vi "Fit VI window to Visible Content.vi"(4 "error in (no error)":errorcluster, 6 "border spacing (2 px)":i32=2, 7 "VI Ref (calling VI)":refnum<vi>) -> (0 "error out":errorcluster, 3 "dup VI Ref":refnum<vi>)   [LabVIEW 2017]
doc: "This utility will fit (resize and center) a VI (defined by the \"VI Ref\" input) about the all of the Front Panel object. It will add a border defined by border spacing in units of pixels. If no VI Reference is passed in, it will operate on the calling VI."
uses:
  <userlib>/_OpenG.lib/appcontrol/appcontrol.llb/Close Generic Object Refnum (Array)__ogtk.vi
panel:
  # "Fit VI window to Content.vi\n\nFits a VI's front panel window to its FP Contents.\n\nPlease visit http://www.OpenG.org to learn about the\nOpen Source LabVIEW software movement.\n\nNOTICE -- YOU MUST LEAVE THIS NOTICE IN PLACE.  PER THE TERMS OF THE LICENSE BELOW, YOU MAY SUBLICENSE THIS SOFTWARE \nIN ANY WAY THAT DOES NOT CONFLICT WITH THIS LICENSE.\n\n### BSD License (http://www.opensource.org/licenses/bsd-license.php) Begin ###\n \nCopyright (c) 2002-2004, Jim Kring <jim@jimkring.com>\nCopyright (c) 2002, Cal-Bay Systems, Inc. <info@calbay.com>\n\nAll rights reserved.\n\nRedistribution and use in source and binary forms, with or without modification, are permitted provided that the following conditions are met:\n\n    * Redistributions of source code must retain the above copyright notice, this list of conditions and the following disclaimer.\n    * Redistributions in binary form must reproduce the above copyright notice, this list of conditions and the following disclaimer in the \n       documentation and/or other materials provided with the distribution.\n    * Neither the name of SciWare, James Kring, Inc., nor the names of its contributors may be used to endorse or promote products derived \n       from this software without specific prior written permission.\n\nTHIS SOFTWARE IS PROVIDED BY THE COPYRIGHT HOLDERS AND CONTRIBUTORS \"AS IS\" AND ANY EXPRESS OR IMPLIED WARRANTIES, \nINCLUDING, BUT NOT LIMITED TO, THE IMPLIED WARRANTIES OF MERCHANTABILITY AND FITNESS FOR A PARTICULAR PURPOSE ARE \nDISCLAIMED. IN NO EVENT SHALL THE COPYRIGHT OWNER OR CONTRIBUTORS BE LIABLE FOR ANY DIRECT, INDIRECT, INCIDENTAL,\n SPECIAL, EXEMPLARY, OR CONSEQUENTIAL DAMAGES (INCLUDING, BUT NOT LIMITED TO, PROCUREMENT OF SUBSTITUTE GOODS OR \nSERVICES; LOSS OF USE, DATA, OR PROFITS; OR BUSINESS INTERRUPTION) HOWEVER CAUSED AND ON ANY THEORY OF LIABILITY, \nWHETHER IN CONTRACT, STRICT LIABILITY, OR TORT (INCLUDING NEGLIGENCE OR OTHERWISE) ARISING IN ANY WAY OUT OF THE USE \nOF THIS SOFTWARE, EVEN IF ADVISED OF THE POSSIBILITY OF SUCH DAMAGE.\n\n### BSD License End ###"
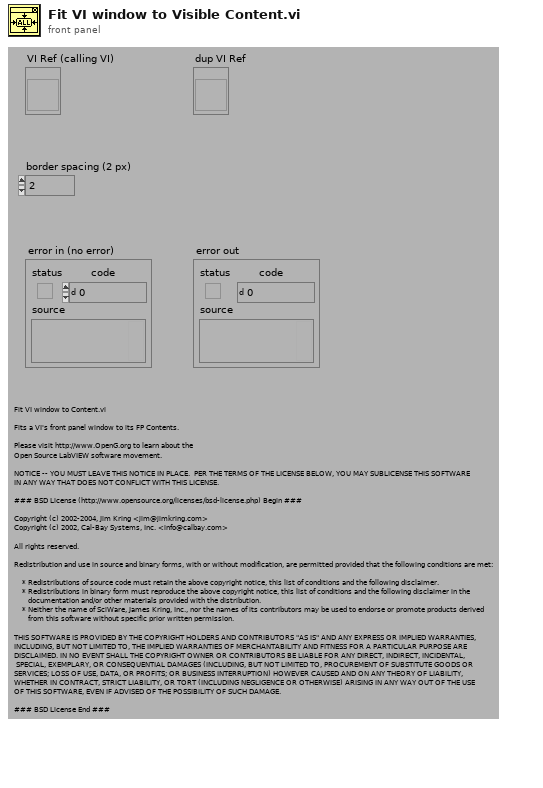
[diagram p1: front panel]
types:
  T1 = typedef "LVRectTypeDef.ctl" = cluster{"Left":i16, "Top":i16, "Right":i16, "Bottom":i16}
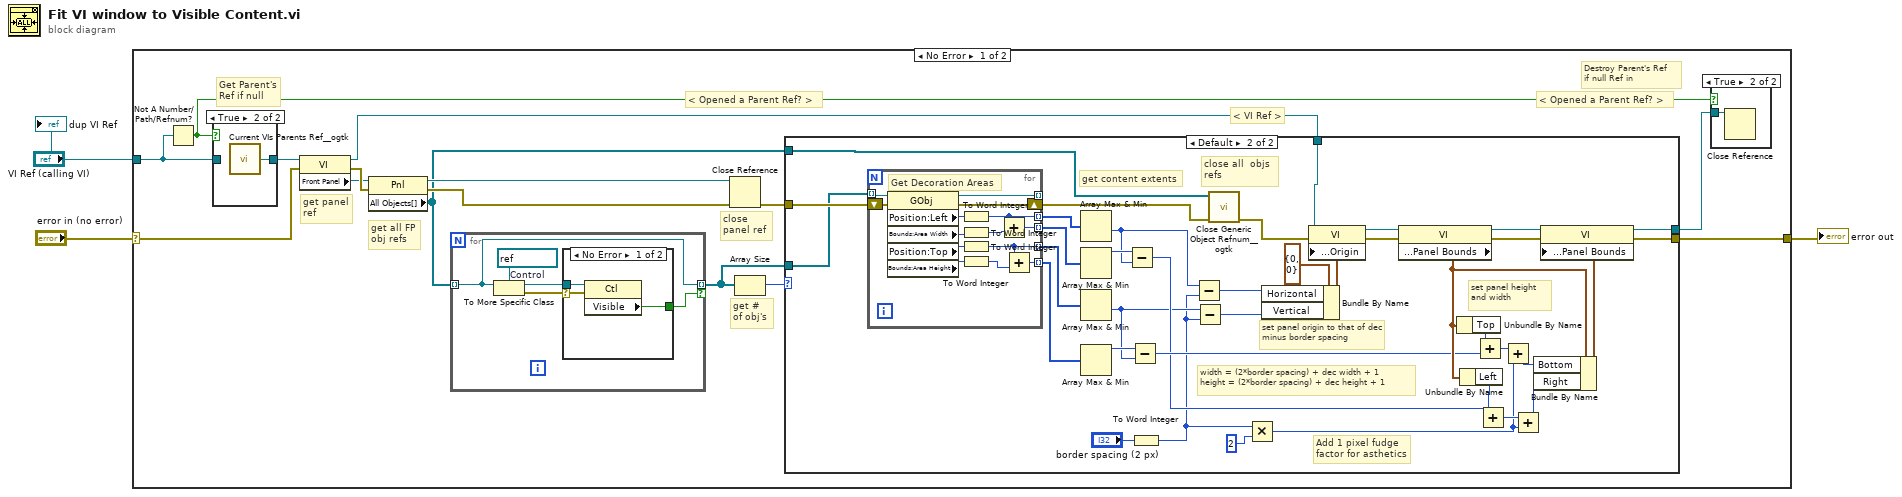
[diagram p0: block diagram]
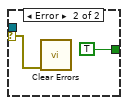
[diagram p2: hidden frame]
diagram:
  n1 = case shown="No Error" "error in (no error)" {
    selector: "error in (no error)" -> [w6 w86]
    tunnel: [w12 w86] -> w3
    tunnel: "VI Ref (calling VI)" -> [w7 _]
    frame No Error {
      # "< Opened a Parent Ref? >"
      # "< Opened a Parent Ref? >"
      # "Destroy Parent's Ref\nif null Ref in"
      # "Get Parent's\nRef if null"
      # "get # of obj's"
      # "get panel ref"
      # "get all FP obj refs"
      # "close panel ref"
      # "< VI Ref >"
      n2 = Not A Number/Path/Refnum?(number/path/refnum=w7) -> (NaN/Path/Refnum?=w9:bool)
      n3 = case shown="True" w9 {
        tunnel: [w30 w31] -> w10
        tunnel: w7 -> [w30 _]
        frame False {
        }
        frame True {
          n4 = call <userlib>:"Current VIs Parents Ref__ogtk.vi"() -> ("Calling VI's Reference"=w31:refnum<vi>)  [unwired: 2 in]
        }
      }
      n5 = property on="Property Node" class="VI"(reference=w10, error in=w6) -> (reference out=w18:refnum<vi>, error out=w16:errorcluster, "Front Panel"=w14:refnum<vi>)
      n6 = property on="Property Node" class="Pnl"(reference=w14, error in=w16) -> (reference out=w17:refnum<vi>, error out=w15:errorcluster, "All Objects[]"=w5:refnum<vi>[])
      n7 = for {
        tunnel: [w19] -> w4 mode=indexing if=w20
        tunnel: w5 -> [w19] mode=indexing
        w22 = refnum<vi> refnum  # Control
        n8 = To More Specific Class(target class=w22, reference=w19) -> (specific class reference=w23:refnum<vi>, error out=w21:errorcluster)  [unwired: 1 in]
        n9 = case shown="No Error" w21 {
          selector: w21 -> [w25 w27]
          tunnel: w23 -> [w26 _]
          tunnel: [w24 TRUE ("Visible")] -> w20
          frame No Error {
            n10 = property class="Ctl"(reference=w26, error in=w25) -> ("Visible"=w24:bool)  [unwired: 2 out]
          }
          frame Error {
            n11 = call <vilib>:"Clear Errors.vi"("error in (no error)"=w27) -> ()  [unwired: 5 in, 2 out]
          }
        }
      }
      n12 = Close Reference(reference=w17, error in (no error)=w15) -> (error out=w13:errorcluster)
      n13 = Array Size(array=w4) -> (size(s)=w11:i32)
      n14 = case shown="Default" w11 {
        tunnel: w18 -> [w33 w69]
        tunnel: w13 -> [w32 w56]
        tunnel: [w32 w51] -> w12
        tunnel: [w33 w50] -> w8
        tunnel: w5 -> [_ w35]
        tunnel: w4 -> [_ w34]
        frame 0 {
          # "do nothing if no objects"
        }
        frame Default {
          # "width = (2*border spacing) + dec width + 1\nheight = (2*border spacing) + dec height + 1"
          # "set panel height and width"
          # "set panel origin to that of dec minus border spacing"
          # "close all  objs refs"
          # "get content extents"
          # "Add 1 pixel fudge factor for asthetics"
          n15 = for {
            tunnel: w34 -> [w85] mode=indexing
            shift-right: [w83] -> w38
            shift-left: w56 -> [w84]
            tunnel: [w82] -> _ mode=indexing
            tunnel: [w78] -> w48 mode=indexing
            tunnel: [w80] -> w47 mode=indexing
            tunnel: [w74] -> w46 mode=indexing
            tunnel: [w79] -> w45 mode=indexing
            # "Get Decoration Areas"
            n16 = property class="GObj"(reference=w85, error in=w84) -> (reference out=w82:refnum<vi>, error out=w83:errorcluster, "Position:Left"=w81:i32, "Bounds:Area Width"=w77:u32, "Position:Top"=w75:i32, "Bounds:Area Height"=w73:u32)
            n17 = To Word Integer(number=w81) -> (16bit integer=w78:i16)
            n18 = To Word Integer(number=w77) -> (16bit integer=w76:i16)
            n19 = To Word Integer(number=w75) -> (16bit integer=w74:i16)
            n20 = To Word Integer(number=w73) -> (16bit integer=w72:i16)
            n21 = Add(x=w78, y=w76) -> (x+y=w80:i16)
            n22 = Add(x=w74, y=w72) -> (x+y=w79:i16)
          }
          n23 = Array Max & Min(array=w48) -> (min value=w39:i16)  [unwired: 3 out]
          n24 = Array Max & Min(array=w47) -> (max value=w42:i16)  [unwired: 3 out]
          n25 = Array Max & Min(array=w46) -> (min value=w40:i16)  [unwired: 3 out]
          n26 = Array Max & Min(array=w45) -> (max value=w44:i16)  [unwired: 3 out]
          n27 = Subtract(x=w42, y=w39) -> (x-y=w41:i16)
          n28 = Subtract(x=w44, y=w40) -> (x-y=w43:i16)
          n29 = To Word Integer(number="border spacing (2 px)") -> (16bit integer=w36:i16)
          n30 = Subtract(x=w39, y=w36) -> (x-y=w59:i16)
          n31 = Subtract(x=w40, y=w36) -> (x-y=w60:i16)
          n32 = call-poly <userlib>:"Close Generic Object Refnum__ogtk.vi"("error in (no error)"=w38, "Gen Refnum Array"=w35) -> ("error out"=w37:errorcluster)  [unwired: 9 in]
          n33 = Multiply(x=w36, y=i16 2) -> (x*y=w49:i16)
          n34 = Bundle By Name(cluster=cluster{"Horizontal":i16, "Vertical":i16} {"Horizontal"=0, "Vertical"=0} ("Front Panel Window:Origin"), "Horizontal"=w59, "Vertical"=w60) -> (w57:cluster{"Horizontal":i16, "Vertical":i16})
          n35 = property on="Property Node" class="VI"(reference=w69, error in=w37, "Front Panel Window:Origin"=w57) -> (reference out=w70:refnum<vi>, error out=w53:errorcluster)
          n36 = property on="Property Node" class="VI"(reference=w70, error in=w53) -> (reference out=w71:refnum<vi>, error out=w52:errorcluster, "Front Panel Window:Panel Bounds"=w61:T1)
          n37 = Unbundle By Name(w61) -> ("Top"=w62:i16)
          n38 = Unbundle By Name(w61) -> ("Left"=w63:i16)
          n39 = Add(x=w62, y=w43) -> (x+y=w67:i16)
          n40 = Add(x=w63, y=w41) -> (x+y=w65:i16)
          n41 = Add(x=w67, y=w49) -> (x+y=w68:i16)
          n42 = Add(x=w65, y=w49) -> (x+y=w66:i16)
          n43 = Bundle By Name(cluster=w61, "Bottom"=w68, "Right"=w66) -> (w64:T1)
          n44 = property on="Property Node" class="VI"(reference=w71, error in=w52, "Front Panel Window:Panel Bounds"=w64) -> (reference out=w50:refnum<vi>, error out=w51:errorcluster)
        }
      }
      n45 = case shown="True" w9 {
        tunnel: w8 -> [_ w29]
        frame False {
        }
        frame True {
          n46 = Close Reference(reference=w29) -> ()  [unwired: 1 in, 1 out]
        }
      }
    }
    frame Error {
    }
  }
  "error out" <- w3
  "dup VI Ref" <- "VI Ref (calling VI)"
